vi "题目1.vi"() -> ()   [LabVIEW 2017]
uses:
  <vilib>/measure/NI_MABase.lvlib
panel:
  in  "布尔":bool
  in  "phase 2":dbl caption="相位" format="%.2p"
  in  "amplitude 2":dbl=1.0 caption="幅值" format="%0.2p"
  in  "frequency 2":dbl=10.0 caption="频率" format="%0.2p"
  in  "phase":dbl caption="相位" format="%.2p"
  in  "amplitude":dbl=1.0 caption="幅值" format="%0.2p"
  in  "frequency":dbl=10.0 caption="频率" format="%0.2p"
  out "波形图 2":waveform(dbl)(graph)
  out "波形图":waveform(dbl)(graph)
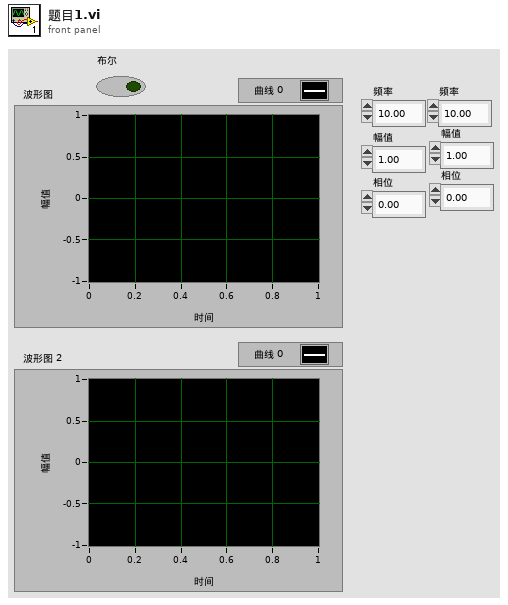
[diagram p1: front panel]
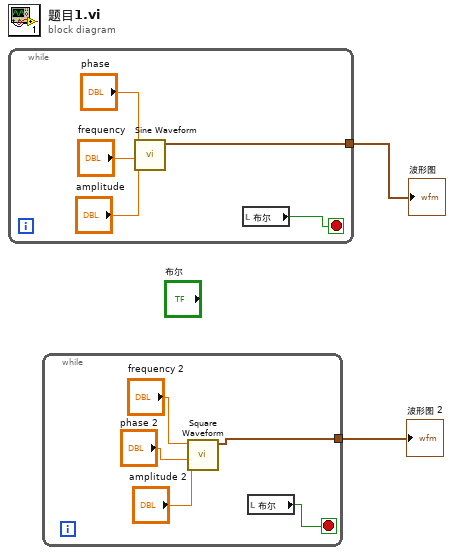
[diagram p0: block diagram]
diagram:
  n1 = while {
    tunnel: [w7] -> w2
    stop <- w3 stop-if-true
    n2 = call <vilib>:"Sine Waveform.vi"("phase"="phase", "amplitude"="amplitude", "frequency"="frequency") -> ("signal out"=w7:waveform(dbl))  [unwired: 7 in, 1 out]
    n3 = local read "布尔"() -> (w3:bool)
  }
  "波形图" <- w2
  n4 = while {
    tunnel: [w12] -> w1
    stop <- w8 stop-if-true
    n5 = call <vilib>:"Square Waveform.vi"("phase"="phase 2", "amplitude"="amplitude 2", "frequency"="frequency 2") -> ("signal out"=w12:waveform(dbl))  [unwired: 7 in, 1 out]
    n6 = local read "布尔"() -> (w8:bool)
  }
  "波形图 2" <- w1
